vi "RT-target - single rate.vi"() -> ()   [LabVIEW 2020]
uses:
  <vilib>/RioEmbeddedCAN/RioEmbeddedCAN.llb/CANFrameControl.ctl
panel:
  out "Delay (ms)":u32
  out "Iteration":i32
  out "CAN input":T1
  out "CAN output":T2 {"type" items=["CAN Data", "CAN Remote"]; "identifier" format="%.0x"}
  in  "stop":bool
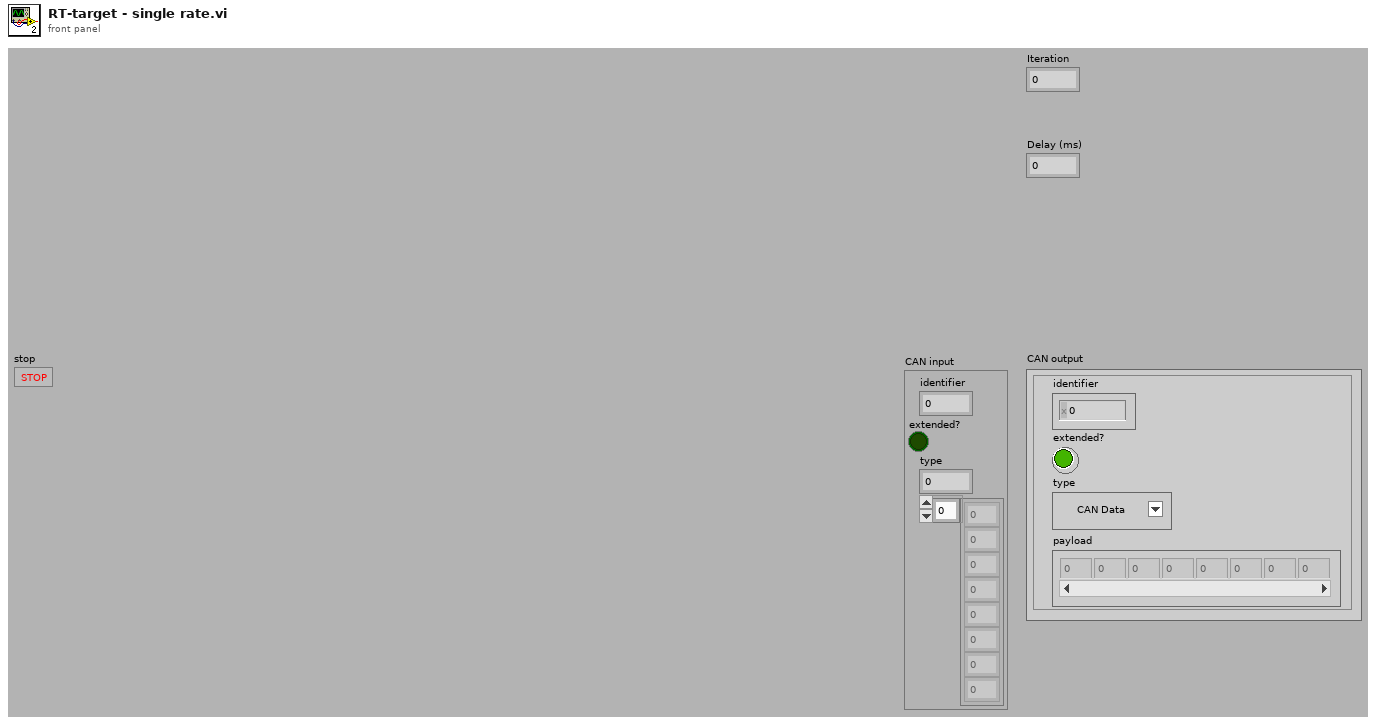
[diagram p1: front panel]
types:
  T1 = cluster{"identifier":u32, "extended?":bool, "type":u8, u64[]}
  T2 = typedef "CANFrameControl.ctl" = cluster{"identifier":u32, "extended?":bool, "type":u8, "payload":u8[]}
  T3 = cluster{"Weights (1000x2001)":dbl[][], "Weights (4x4x1000x15)":dbl[][][][], "Weights (4x4x15x8)":dbl[][][][], "Weights (4x9)":dbl[][]}
  T4 = cluster{"FPGA VI Reference Out":refnum<k20>, "error out":errorcluster}
  T5 = cluster{"Boolean":bool, "initialized array":string[][], "interface object out":refnum<k20>, "error out":errorcluster}
  T6 = cluster{"interface object out":refnum<k20>, "error out":errorcluster}
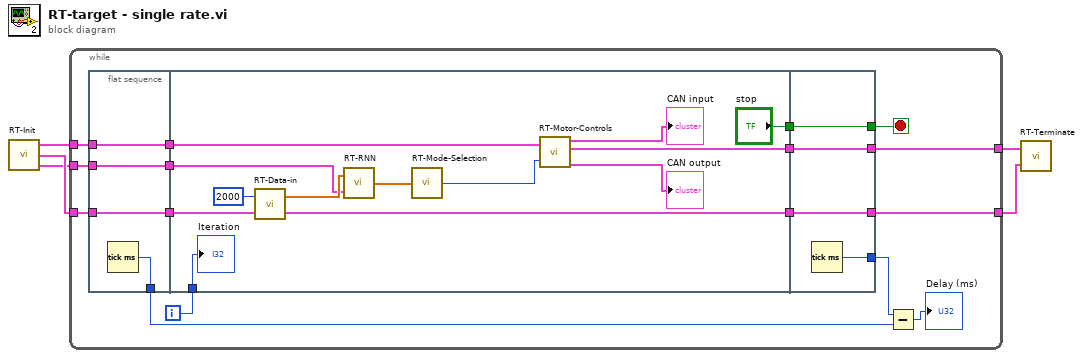
[diagram p0: block diagram]
diagram:
  n1 = call "RT-Init.vi"() -> ("Weights"=w3:T3, "Data-in Settings"=w5:T4, "Motor-Controller Settings"=w4:T5)
  n2 = while {
    tunnel: w5 -> [w20]
    tunnel: w4 -> [w19]
    tunnel: [w18] -> w1
    tunnel: [w17] -> w2
    tunnel: w3 -> [w16]
    i -> [w15]
    stop <- w21 stop-if-true
    n3 = flat-sequence {
      tunnel: w16 -> [w23]
      tunnel: w19 -> [w24]
      tunnel: w20 -> [w25]
      tunnel: [w25] -> w14
      tunnel: [w24] -> w13
      tunnel: [w23] -> w12
      tunnel: [w22] -> w6
      tunnel: w15 -> [w26]
      tunnel: w14 -> [w34]
      tunnel: w13 -> [w33]
      tunnel: w12 -> [w28]
      tunnel: ["stop"] -> w11
      tunnel: [w32] -> w10
      tunnel: [w31] -> w9
      tunnel: [w40] -> w17
      tunnel: [w41] -> w18
      tunnel: [w42] -> w21
      tunnel: w11 -> [w42]
      tunnel: w10 -> [w41]
      tunnel: w9 -> [w40]
      tunnel: [w39] -> w7
      frame #0 {
        n4 = Tick Count (ms)() -> (millisecond timer value=w22:u32)
      }
      frame #1 {
        n5 = call "RT-Data-in.vi"("cluster"=w34, "Amount of Inputs"=2000) -> ("Error"=w31:T4, "Bicep+Triceps"=w38:dbl[])
        n6 = call "RT-RNN.vi"("Weights Cluster"=w28, "Input"=w38) -> ("Output"=w30:dbl[])
        n7 = call "RT-Mode-Selection.vi"("Array"=w30) -> ("U64-Output"=w29:u64)
        n8 = call "RT-Motor-Controls.vi"("Settings"=w33, "U64-Input"=w29) -> ("CAN input"=→"CAN input":T1, "Error"=w32:T6, "CAN output"=→"CAN output":T2)  [unwired: 1 in]
        "Iteration" <- w26
      }
      frame #2 {
        n9 = Tick Count (ms)() -> (millisecond timer value=w39:u32)
      }
    }
    n10 = Subtract(x=w7, y=w6) -> (x-y=→"Delay (ms)":u32)
  }
  n11 = call "RT-Terminate.vi"("Data input"=w2, "Motor Controller"=w1) -> ()  [unwired: 1 in]
